vi "Plot 2 Graph.vi"(4 "VoltDevider":dbl=10.0, 5 "Type":enum16{"All", "Force U+D", "Volt U+D"}(ring), 6 "EnableSmooth":bool, 7 "FillZeroFirstSignal":i32=5, 8 "Analog Up":T1={"Angle Data"=[0.0, 1.0, 2.0, 3.0, 4.0, 5.0, 6.0, 7.0, 8.0, 9.0, 10.0, 11.0, 12.0, 13.0, 14.0, 15.0, 16.0, 17.0, 18.0, 19.0, 20.0], "Force Up FW"=[0.0, 0.0, 0.0, 0.01, 0.01, 0.0, 0.01, 0.01, 0.02, 0.022, 0.03, 0.05, 0.07, 0.1, 0.3, 0.55, 0.67, 0.85, 0.92, 1.15, 1.2], "Force Up RW"=[0.0, 0.0, 0.0, 0.01, 0.01, 0.0, 0.01, 0.01, 0.02, 0.022, 0.03, 0.05, 0.07, 0.1, 0.3, 0.55, 0.67, 0.85, 0.92, 1.15, 1.2], "Volt 1 FW"=[0.0, 0.0, 0.0, 0.0, 0.0, 0.0, 0.0, 0.1, 0.0, 0.0, 0.0, 0.1, 0.0, 0.3, 0.4, 0.5, 0.5, 12.0, 12.0, 12.0, 12.0], "Volt 1 RW"=[0.0, 0.0, 0.0, 0.0, 0.0, 0.0, 0.0, 0.0, 0.0, 0.0, 0.0, 0.0, 0.0, 0.0, 0.0, 0.0, 0.0, 0.0, 0.0, 0.0, 0.0], "Volt 2 FW"=[0.0, 0.0, 0.0, 0.0, 0.0, 0.0, 0.0, 0.0, 0.0, 0.0, 0.0, 0.0, 0.0, 0.0, 0.0, 0.0, 0.0, 0.0, 0.0, 0.0, 0.0], "Volt 2 RW"=[0.0, 0.0, 0.0, 0.0, 0.0, 0.0, 0.0, 0.0, 0.0, 0.0, 0.0, 0.0, 0.0, 0.0, 0.0, 0.0, 0.0, 0.0, 0.0, 0.0, 0.0]}, 11 "Analog Down":T2={"Angle Data"=[0.0, 1.0, 2.0, 3.0, 4.0, 5.0, 6.0, 7.0, 8.0, 9.0, 10.0, 11.0, 12.0, 13.0, 14.0, 15.0, 16.0, 17.0, 18.0, 19.0, 20.0], "Force Down FW"=[0.0, 0.1, 0.2, 0.25, 0.3, 0.35, 0.4, 0.45, 0.49, 0.48, 0.5, 0.55, 0.58, 0.7, 0.935, 1.1, 1.125, 1.17, 1.18, 1.19, 1.2], "Force Down RW"=[0.0, 0.1, 0.2, 0.25, 0.3, 0.35, 0.4, 0.45, 0.49, 0.48, 0.5, 0.55, 0.58, 0.7, 0.935, 1.1, 1.125, 1.17, 1.18, 1.19, 1.2], "Volt 1 FW"=[0.0, 0.0, 0.0, 0.0, 0.0, 0.0, 0.1, 0.1, 0.0, 0.0, 0.0, 0.0, 0.3, 12.0, 12.0, 12.0, 12.0, 12.0, 12.0, 12.0, 12.0], "Volt 1 RW"=[0.0, 0.0, 0.1, 0.0, 0.0, 0.0, 0.0, 0.0, 0.1, 0.0, 0.0, 0.1, 0.0, 0.0, 0.0, 0.2, 0.0, 0.0, 0.0, 0.0, 0.0], "Volt 2 FW"=[0.0, 0.0, 0.0, 0.0, 0.0, 0.0, 0.0, 0.0, 0.0, 0.0, 0.0, 0.0, 0.0, 0.0, 0.0, 0.0, 0.0, 0.0, 0.0, 0.0, 0.0], "Volt 2 RW"=[0.0, 0.0, 0.0, 0.0, 0.0, 0.0, 0.0, 0.0, 0.0, 0.0, 0.0, 0.0, 0.0, 0.0, 0.0, 0.0, 0.0, 0.0, 0.0, 0.0, 0.0]}) -> (0 "XY Up":cluster{"Angle Data":dbl[], "Array":dbl[]}[](graph), 3 "XY Down":cluster{"Angle Data":dbl[], "Array":dbl[]}[](graph))   [LabVIEW 2017]
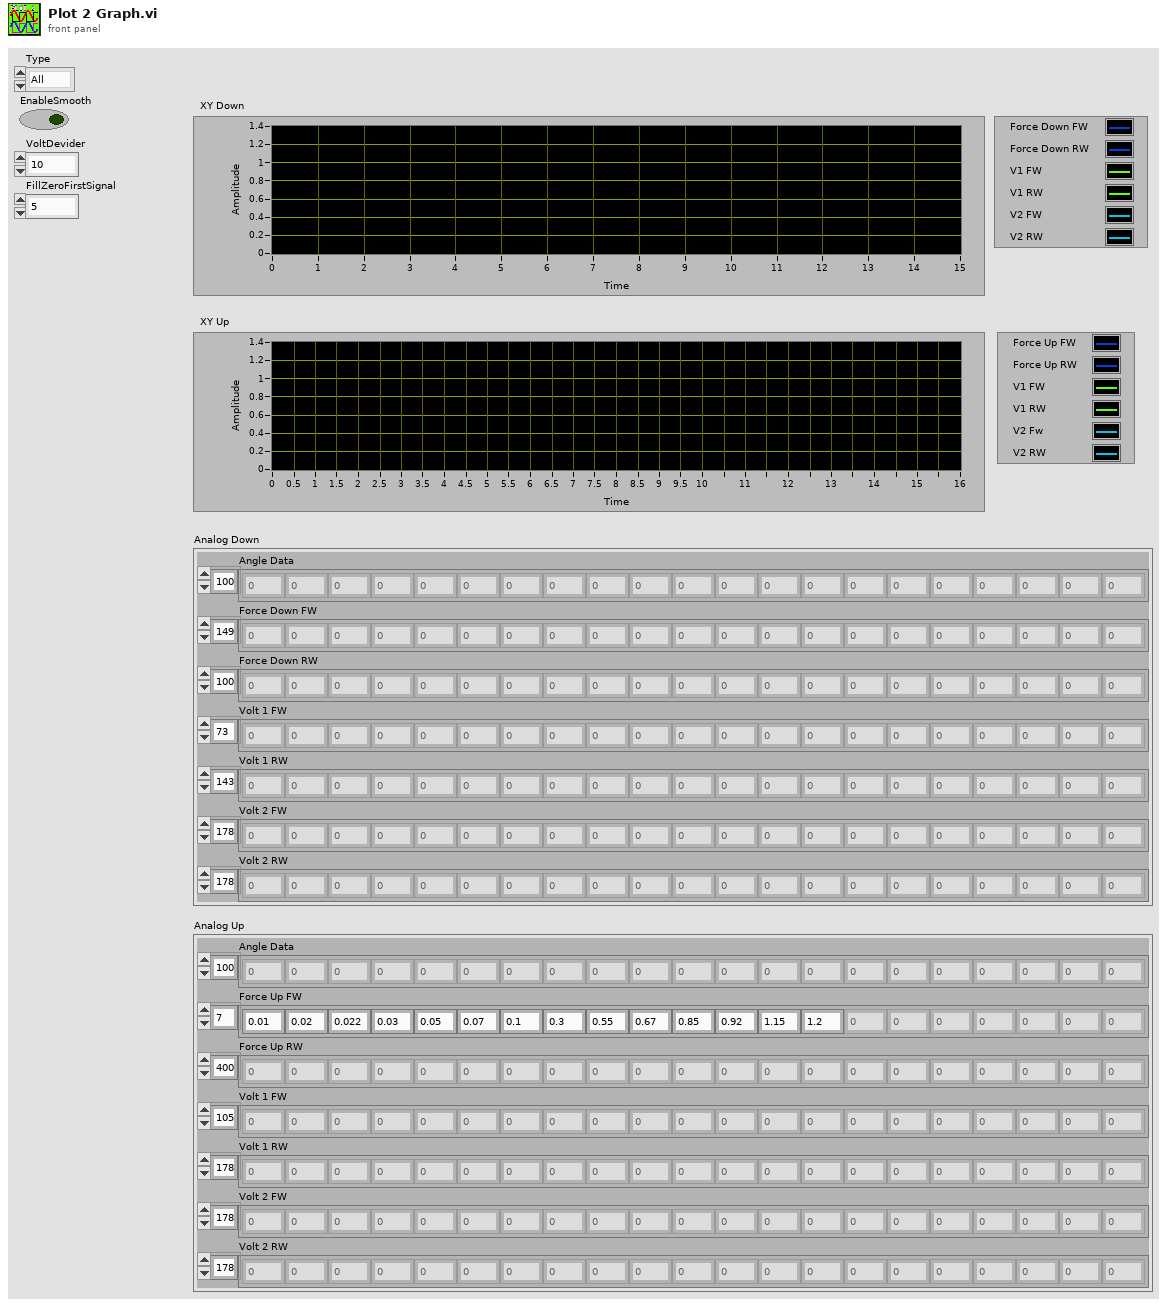
[diagram p1: front panel]
types:
  T1 = cluster{"Angle Data":dbl[], "Force Up FW":dbl[], "Force Up RW":dbl[], "Volt 1 FW":dbl[], "Volt 1 RW":dbl[], "Volt 2 FW":dbl[], "Volt 2 RW":dbl[]}
  T2 = cluster{"Angle Data":dbl[], "Force Down FW":dbl[], "Force Down RW":dbl[], "Volt 1 FW":dbl[], "Volt 1 RW":dbl[], "Volt 2 FW":dbl[], "Volt 2 RW":dbl[]}
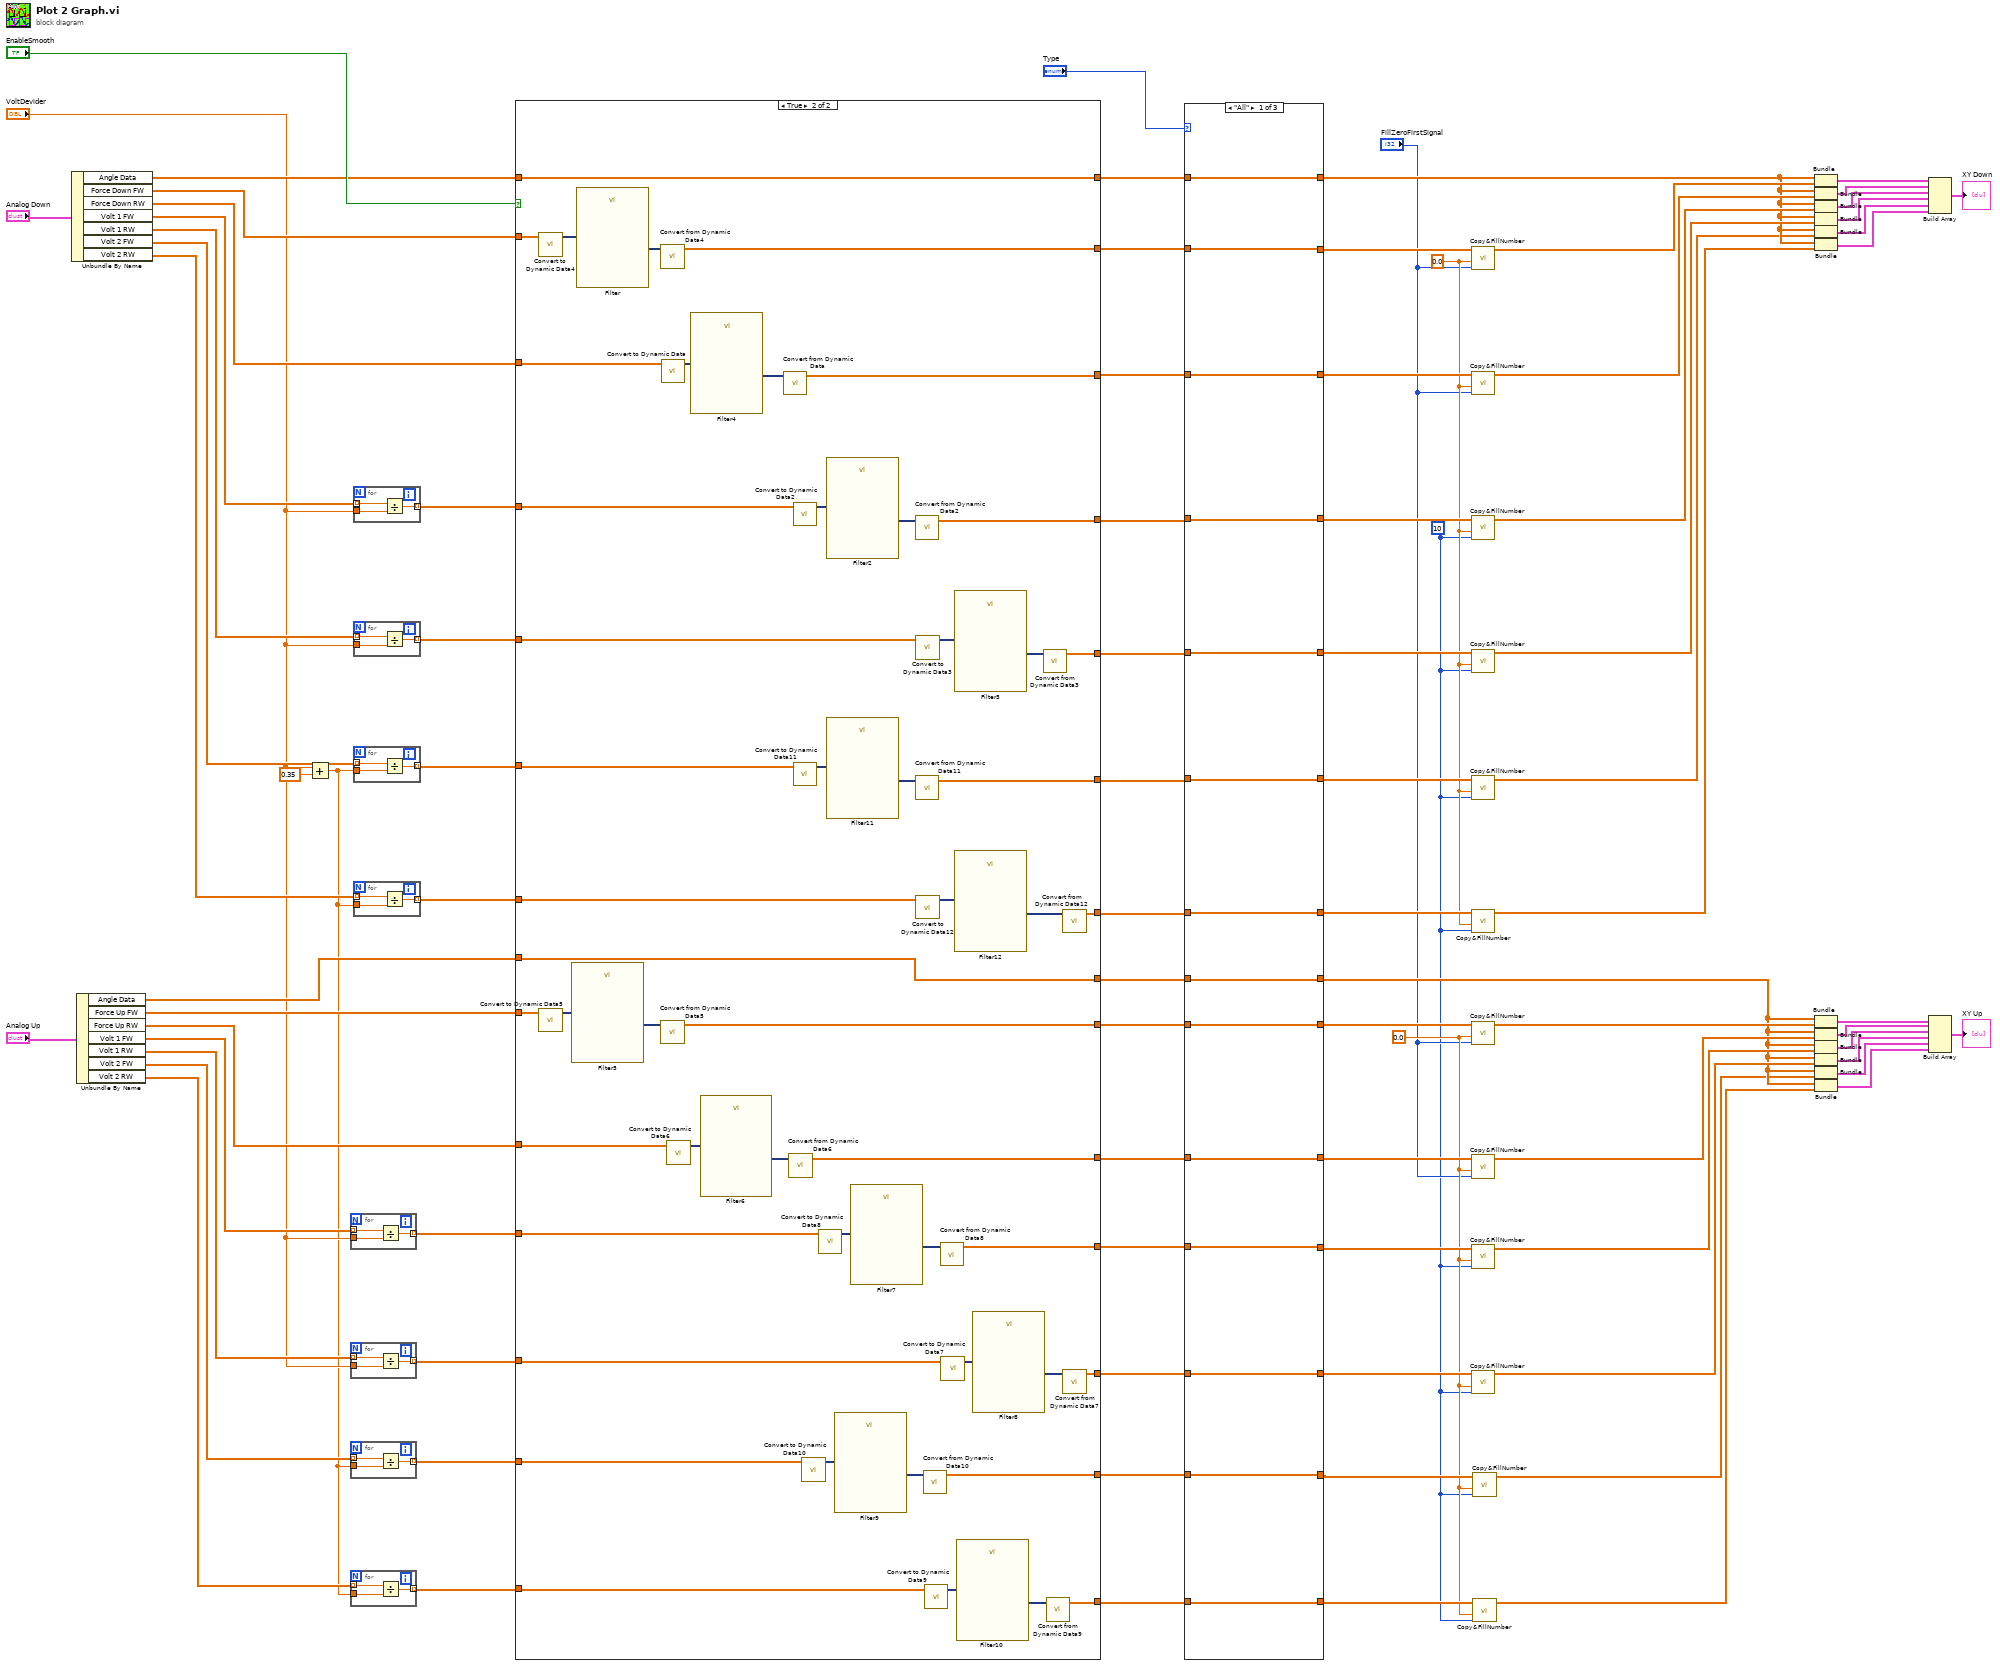
[diagram p0: block diagram]
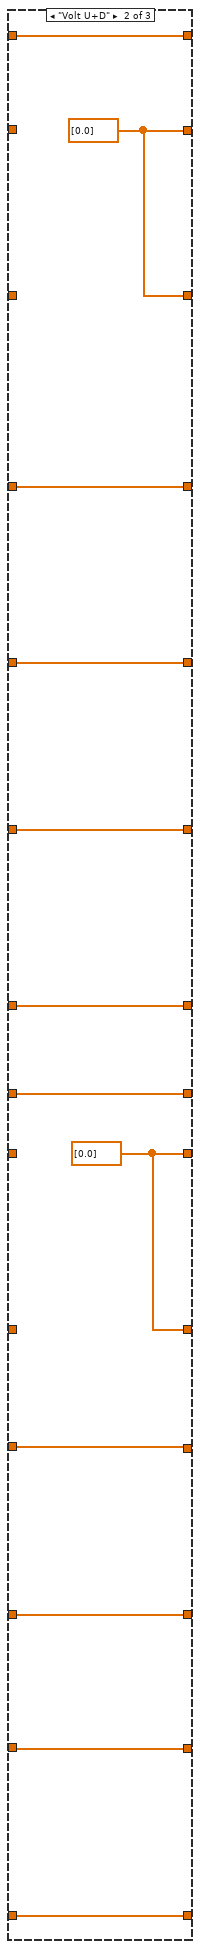
[diagram p2: hidden frame]
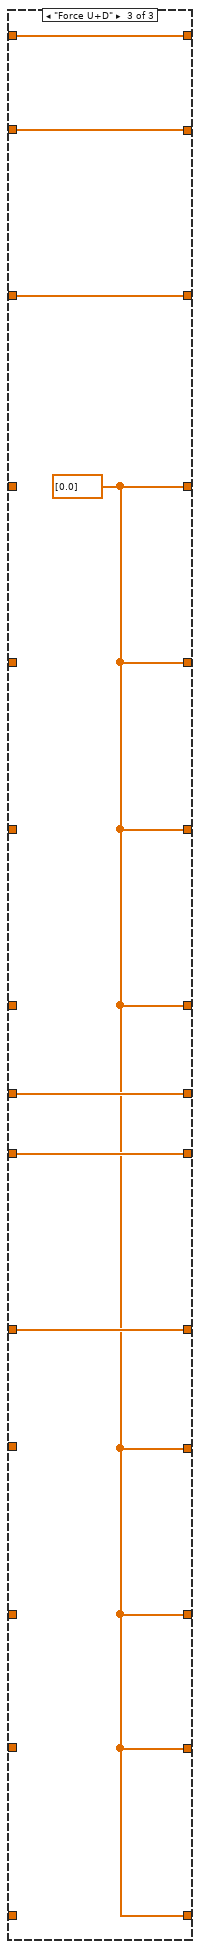
[diagram p3: hidden frame]
diagram:
  w1 = 10 ("Length")
  w3 = 0.0 ("Level In")
  w12 = 0.0 ("Level In")
  n1 = Unbundle By Name("Analog Down") -> ("Angle Data"=w37:dbl[], "Force Down FW"=w77:dbl[], "Force Down RW"=w52:dbl[], "Volt 1 FW"=w51:dbl[], "Volt 1 RW"=w50:dbl[], "Volt 2 FW"=w14:dbl[], "Volt 2 RW"=w13:dbl[])
  n2 = Unbundle By Name("Analog Up") -> ("Angle Data"=w35:dbl[], "Force Up FW"=w44:dbl[], "Force Up RW"=w43:dbl[], "Volt 1 FW"=w41:dbl[], "Volt 1 RW"=w39:dbl[], "Volt 2 FW"=w33:dbl[], "Volt 2 RW"=w32:dbl[])
  n3 = Add(x="VoltDevider", y=0.35) -> (x+y=w4:dbl)
  n4 = for {
    tunnel: [w90] -> w42 mode=indexing
    tunnel: "VoltDevider" -> [w89]
    tunnel: w41 -> [w88] mode=indexing
    n5 = Divide(x=w88, y=w89) -> (x/y=w90:dbl)
  }
  n6 = for {
    tunnel: [w93] -> w40 mode=indexing
    tunnel: "VoltDevider" -> [w92]
    tunnel: w39 -> [w91] mode=indexing
    n7 = Divide(x=w91, y=w92) -> (x/y=w93:dbl)
  }
  n8 = for {
    tunnel: [w96] -> w31 mode=indexing
    tunnel: w4 -> [w95]
    tunnel: w33 -> [w94] mode=indexing
    n9 = Divide(x=w94, y=w95) -> (x/y=w96:dbl)
  }
  n10 = for {
    tunnel: [w99] -> w30 mode=indexing
    tunnel: w4 -> [w98]
    tunnel: w32 -> [w97] mode=indexing
    n11 = Divide(x=w97, y=w98) -> (x/y=w99:dbl)
  }
  n12 = for {
    tunnel: w51 -> [w102] mode=indexing
    tunnel: [w101] -> w85 mode=indexing
    tunnel: "VoltDevider" -> [w100]
    n13 = Divide(x=w102, y=w100) -> (x/y=w101:dbl)
  }
  n14 = for {
    tunnel: w50 -> [w105] mode=indexing
    tunnel: [w104] -> w84 mode=indexing
    tunnel: "VoltDevider" -> [w103]
    n15 = Divide(x=w105, y=w103) -> (x/y=w104:dbl)
  }
  n16 = for {
    tunnel: w14 -> [w108] mode=indexing
    tunnel: [w107] -> w17 mode=indexing
    tunnel: w4 -> [w106]
    n17 = Divide(x=w108, y=w106) -> (x/y=w107:dbl)
  }
  n18 = for {
    tunnel: w13 -> [w111] mode=indexing
    tunnel: [w110] -> w18 mode=indexing
    tunnel: w4 -> [w109]
    n19 = Divide(x=w111, y=w109) -> (x/y=w110:dbl)
  }
  n20 = case shown="True" "EnableSmooth" {
    tunnel: [w123 w175] -> w83
    tunnel: [w124 w172] -> w82
    tunnel: [w125 w171] -> w81
    tunnel: w85 -> [w124 w174]
    tunnel: w84 -> [w125 w173]
    tunnel: [w121 w170] -> w80
    tunnel: w52 -> [w123 w169]
    tunnel: w77 -> [w121 w168]
    tunnel: [w119 w163] -> w75
    tunnel: [w118 w162] -> w76
    tunnel: [w117 w161] -> w71
    tunnel: [w116 w160] -> w70
    tunnel: w44 -> [w119 w155]
    tunnel: w43 -> [w118 w154]
    tunnel: w42 -> [w117 w153]
    tunnel: w40 -> [w116 w152]
    tunnel: w37 -> [w122 w151]
    tunnel: [w122 w151] -> w38
    tunnel: [w120 w150] -> w36
    tunnel: w35 -> [w120 w150]
    tunnel: w31 -> [w115 w149]
    tunnel: w30 -> [w114 w148]
    tunnel: [w115 w147] -> w29
    tunnel: [w114 w146] -> w28
    tunnel: w17 -> [w113 w143]
    tunnel: w18 -> [w112 w142]
    tunnel: [w113 w145] -> w16
    tunnel: [w112 w144] -> w15
    frame False {
    }
    frame True {
      n21 = call "Convert to Dynamic Data4"("Array"=w168) -> ("Dynamic Data Type"=w159:dynamicdata)  [unwired: 3 in]
      n22 = call "Convert to Dynamic Data5"("Array"=w155) -> ("Dynamic Data Type"=w165:dynamicdata)  [unwired: 3 in]
      n23 = call "Filter5"("Signal"=w165) -> ("Filtered Signal"=w164:dynamicdata)  [unwired: 9 in, 1 out]
      n24 = call "Filter"("Signal"=w159) -> ("Filtered Signal"=w158:dynamicdata)  [unwired: 9 in, 1 out]
      n25 = call "Convert from Dynamic Data4"("Dynamic Data Type"=w158) -> ("Array"=w170:dbl[])  [unwired: 3 in]
      n26 = call "Convert from Dynamic Data5"("Dynamic Data Type"=w164) -> ("Array"=w163:dbl[])  [unwired: 3 in]
      n27 = call "Convert to Dynamic Data"("Array"=w169) -> ("Dynamic Data Type"=w157:dynamicdata)  [unwired: 3 in]
      n28 = call "Convert to Dynamic Data6"("Array"=w154) -> ("Dynamic Data Type"=w166:dynamicdata)  [unwired: 3 in]
      n29 = call "Filter4"("Signal"=w157) -> ("Filtered Signal"=w156:dynamicdata)  [unwired: 9 in, 1 out]
      n30 = call "Filter6"("Signal"=w166) -> ("Filtered Signal"=w167:dynamicdata)  [unwired: 9 in, 1 out]
      n31 = call "Convert from Dynamic Data"("Dynamic Data Type"=w156) -> ("Array"=w175:dbl[])  [unwired: 3 in]
      n32 = call "Convert from Dynamic Data6"("Dynamic Data Type"=w167) -> ("Array"=w162:dbl[])  [unwired: 3 in]
      n33 = call "Convert to Dynamic Data2"("Array"=w174) -> ("Dynamic Data Type"=w132:dynamicdata)  [unwired: 3 in]
      n34 = call "Convert to Dynamic Data11"("Array"=w143) -> ("Dynamic Data Type"=w127:dynamicdata)  [unwired: 3 in]
      n35 = call "Convert to Dynamic Data10"("Array"=w149) -> ("Dynamic Data Type"=w134:dynamicdata)  [unwired: 3 in]
      n36 = call "Convert to Dynamic Data8"("Array"=w153) -> ("Dynamic Data Type"=w141:dynamicdata)  [unwired: 3 in]
      n37 = call "Filter2"("Signal"=w132) -> ("Filtered Signal"=w133:dynamicdata)  [unwired: 9 in, 1 out]
      n38 = call "Filter11"("Signal"=w127) -> ("Filtered Signal"=w126:dynamicdata)  [unwired: 9 in, 1 out]
      n39 = call "Filter9"("Signal"=w134) -> ("Filtered Signal"=w135:dynamicdata)  [unwired: 9 in, 1 out]
      n40 = call "Filter7"("Signal"=w141) -> ("Filtered Signal"=w140:dynamicdata)  [unwired: 9 in, 1 out]
      n41 = call "Convert from Dynamic Data2"("Dynamic Data Type"=w133) -> ("Array"=w172:dbl[])  [unwired: 3 in]
      n42 = call "Convert from Dynamic Data11"("Dynamic Data Type"=w126) -> ("Array"=w145:dbl[])  [unwired: 3 in]
      n43 = call "Convert to Dynamic Data3"("Array"=w173) -> ("Dynamic Data Type"=w131:dynamicdata)  [unwired: 3 in]
      n44 = call "Convert to Dynamic Data12"("Array"=w142) -> ("Dynamic Data Type"=w128:dynamicdata)  [unwired: 3 in]
      n45 = call "Convert from Dynamic Data10"("Dynamic Data Type"=w135) -> ("Array"=w147:dbl[])  [unwired: 3 in]
      n46 = call "Convert to Dynamic Data9"("Array"=w148) -> ("Dynamic Data Type"=w136:dynamicdata)  [unwired: 3 in]
      n47 = call "Convert from Dynamic Data8"("Dynamic Data Type"=w140) -> ("Array"=w161:dbl[])  [unwired: 3 in]
      n48 = call "Convert to Dynamic Data7"("Array"=w152) -> ("Dynamic Data Type"=w139:dynamicdata)  [unwired: 3 in]
      n49 = call "Filter3"("Signal"=w131) -> ("Filtered Signal"=w130:dynamicdata)  [unwired: 9 in, 1 out]
      n50 = call "Filter12"("Signal"=w128) -> ("Filtered Signal"=w129:dynamicdata)  [unwired: 9 in, 1 out]
      n51 = call "Filter10"("Signal"=w136) -> ("Filtered Signal"=w137:dynamicdata)  [unwired: 9 in, 1 out]
      n52 = call "Filter8"("Signal"=w139) -> ("Filtered Signal"=w138:dynamicdata)  [unwired: 9 in, 1 out]
      n53 = call "Convert from Dynamic Data3"("Dynamic Data Type"=w130) -> ("Array"=w171:dbl[])  [unwired: 3 in]
      n54 = call "Convert from Dynamic Data9"("Dynamic Data Type"=w137) -> ("Array"=w146:dbl[])  [unwired: 3 in]
      n55 = call "Convert from Dynamic Data12"("Dynamic Data Type"=w129) -> ("Array"=w144:dbl[])  [unwired: 3 in]
      n56 = call "Convert from Dynamic Data7"("Dynamic Data Type"=w138) -> ("Array"=w160:dbl[])  [unwired: 3 in]
    }
  }
  n57 = case shown="\"All\"" "Type" {
    tunnel: [w183 w198 w202] -> w64
    tunnel: w82 -> [w183 w198 _]
    tunnel: w81 -> [w182 w197 _]
    tunnel: [w182 w197 w202] -> w62
    tunnel: [w184 w201 w207] -> w66
    tunnel: w83 -> [w184 _ w207]
    tunnel: [w185 w201 w208] -> w68
    tunnel: w80 -> [w185 _ w208]
    tunnel: w76 -> [w188 _ w203]
    tunnel: w75 -> [w189 _ w204]
    tunnel: [w189 w196 w204] -> w60
    tunnel: [w188 w196 w203] -> w58
    tunnel: [w187 w195 w202] -> w56
    tunnel: [w186 w194 w202] -> w54
    tunnel: w71 -> [w187 w195 _]
    tunnel: w70 -> [w186 w194 _]
    tunnel: w38 -> [w181 w200 w206]
    tunnel: [w181 w200 w206] -> w11
    tunnel: [w180 w199 w205] -> w25
    tunnel: w36 -> [w180 w199 w205]
    tunnel: [w179 w193 w202] -> w27
    tunnel: w29 -> [w179 w193 _]
    tunnel: [w178 w192 w202] -> w26
    tunnel: w28 -> [w178 w192 _]
    tunnel: [w176 w191 w202] -> w19
    tunnel: w16 -> [w176 w191 _]
    tunnel: w15 -> [w177 w190 _]
    tunnel: [w177 w190 w202] -> w20
    frame "All" {
    }
    frame "Volt U+D" {
      w196 = dbl[] [0.0] ("Array")
      w201 = dbl[] [0.0] ("Array")
    }
    frame "Force U+D" {
      w202 = dbl[] [0.0] ("Array")
    }
  }
  n58 = call "Copy&FillNumber.vi"("Length"="FillZeroFirstSignal", "Level In"=w12, "Array In"=w68) -> ("Array Out"=w67:dbl[])  [unwired: 8 in]
  n59 = call "Copy&FillNumber.vi"("Length"="FillZeroFirstSignal", "Level In"=w12, "Array In"=w66) -> ("Array Out"=w65:dbl[])  [unwired: 8 in]
  n60 = call "Copy&FillNumber.vi"("Length"=w1, "Level In"=w12, "Array In"=w64) -> ("Array Out"=w63:dbl[])  [unwired: 8 in]
  n61 = call "Copy&FillNumber.vi"("Length"=w1, "Level In"=w12, "Array In"=w62) -> ("Array Out"=w61:dbl[])  [unwired: 8 in]
  n62 = call "Copy&FillNumber.vi"("Length"=w1, "Level In"=w12, "Array In"=w19) -> ("Array Out"=w8:dbl[])  [unwired: 8 in]
  n63 = call "Copy&FillNumber.vi"("Length"=w1, "Level In"=w12, "Array In"=w20) -> ("Array Out"=w7:dbl[])  [unwired: 8 in]
  n64 = call "Copy&FillNumber.vi"("Length"="FillZeroFirstSignal", "Level In"=w3, "Array In"=w60) -> ("Array Out"=w59:dbl[])  [unwired: 8 in]
  n65 = call "Copy&FillNumber.vi"("Length"="FillZeroFirstSignal", "Level In"=w3, "Array In"=w58) -> ("Array Out"=w57:dbl[])  [unwired: 8 in]
  n66 = call "Copy&FillNumber.vi"("Length"=w1, "Level In"=w3, "Array In"=w56) -> ("Array Out"=w55:dbl[])  [unwired: 8 in]
  n67 = call "Copy&FillNumber.vi"("Length"=w1, "Level In"=w3, "Array In"=w54) -> ("Array Out"=w53:dbl[])  [unwired: 8 in]
  n68 = call "Copy&FillNumber.vi"("Length"=w1, "Level In"=w3, "Array In"=w27) -> ("Array Out"=w24:dbl[])  [unwired: 8 in]
  n69 = call "Copy&FillNumber.vi"("Length"=w1, "Level In"=w3, "Array In"=w26) -> ("Array Out"=w23:dbl[])  [unwired: 8 in]
  n70 = Bundle("Angle Data"=w11, "Array Out"=w67) -> (w87:cluster{"Angle Data":dbl[], "Array Out":dbl[]})  [unwired: 1 in]
  n71 = Bundle("Angle Data"=w11, "Array Out"=w65) -> (w74:cluster{"Angle Data":dbl[], "Array Out":dbl[]})  [unwired: 1 in]
  n72 = Bundle("Angle Data"=w11, "Array Out"=w63) -> (w73:cluster{"Angle Data":dbl[], "Array Out":dbl[]})  [unwired: 1 in]
  n73 = Bundle("Angle Data"=w11, "Array Out"=w61) -> (w72:cluster{"Angle Data":dbl[], "Array Out":dbl[]})  [unwired: 1 in]
  n74 = Bundle("Angle Data"=w11, "Array Out"=w8) -> (w10:cluster{"Angle Data":dbl[], "Array Out":dbl[]})  [unwired: 1 in]
  n75 = Bundle("Angle Data"=w11, "Array Out"=w7) -> (w9:cluster{"Angle Data":dbl[], "Array Out":dbl[]})  [unwired: 1 in]
  n76 = Bundle("Angle Data"=w25, "Array Out"=w59) -> (w49:cluster{"Angle Data":dbl[], "Array Out":dbl[]})  [unwired: 1 in]
  n77 = Bundle("Angle Data"=w25, "Array Out"=w57) -> (w48:cluster{"Angle Data":dbl[], "Array Out":dbl[]})  [unwired: 1 in]
  n78 = Bundle("Angle Data"=w25, "Array Out"=w55) -> (w47:cluster{"Angle Data":dbl[], "Array Out":dbl[]})  [unwired: 1 in]
  n79 = Bundle("Angle Data"=w25, "Array Out"=w53) -> (w46:cluster{"Angle Data":dbl[], "Array Out":dbl[]})  [unwired: 1 in]
  n80 = Bundle("Angle Data"=w25, "Array Out"=w24) -> (w22:cluster{"Angle Data":dbl[], "Array Out":dbl[]})  [unwired: 1 in]
  n81 = Bundle("Angle Data"=w25, "Array Out"=w23) -> (w21:cluster{"Angle Data":dbl[], "Array Out":dbl[]})  [unwired: 1 in]
  n82 = Build Array(w87, w74, w73, w72, w10, w9) -> (→"XY Down":cluster{"Angle Data":dbl[], "Array Out":dbl[]}[])
  n83 = Build Array(w49, w48, w47, w46, w22, w21) -> (→"XY Up":cluster{"Angle Data":dbl[], "Array Out":dbl[]}[])
